vi "csm_lumikki_instron_stop.vi"() -> (2 "creepRunningOut":bool, 3 "stopOut":bool)   [LabVIEW 2009]
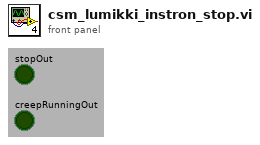
[diagram p1: front panel]
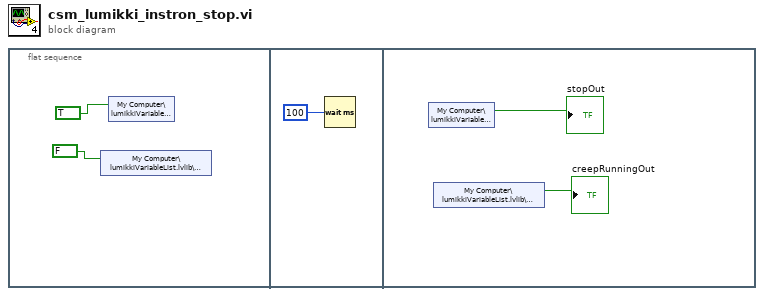
[diagram p0: block diagram]
diagram:
  n1 = flat-sequence {
    frame #0 {
      n2 = shared-variable "My Computer\\lumikkiVariableList.lvlib\\creepRunning"(FALSE ("Busy")) -> ()  [unwired: 1 in, 1 out]
      n3 = shared-variable "My Computer\\lumikkiVariableList.lvlib\\stop"(TRUE ("Busy")) -> ()  [unwired: 1 in, 1 out]
    }
    frame #1 {
      n4 = Wait (ms)(milliseconds to wait=u32 100) -> ()  [unwired: 1 out]
    }
    frame #2 {
      n5 = shared-variable "My Computer\\lumikkiVariableList.lvlib\\stop"() -> (→"stopOut":bool)  [unwired: 1 in, 1 out]
      n6 = shared-variable "My Computer\\lumikkiVariableList.lvlib\\creepRunning"() -> (→"creepRunningOut":bool)  [unwired: 1 in, 1 out]
    }
  }
